vi "Image Data (Raw).vi"(8 "error in (no error)":errorcluster, 11 "Buffer in":refnum<class "Buffer.lvclass">=refnum) -> (0 "error out":errorcluster, 2 "Raw Data":string, 3 "Buffer":refnum<class "Buffer.lvclass">)   [LabVIEW 2020, in "common.lvlib" / "Buffer.lvclass"]
uses:
  Buffer.lvclass
  bin/gindustrialcam_32-1.dll
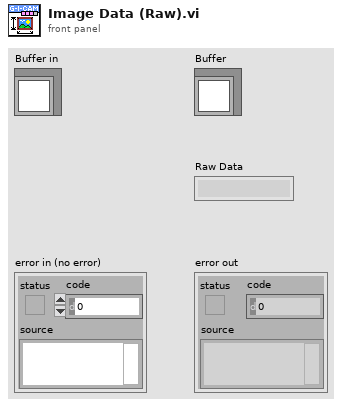
[diagram p1: front panel]
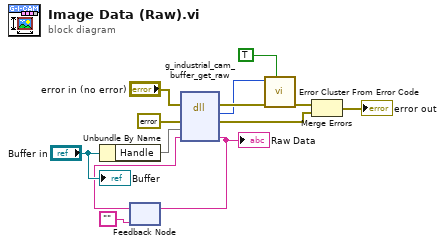
[diagram p0: block diagram]
diagram:
  n1 = Unbundle By Name("Buffer in") -> ("Handle"=w6)
  n2 = feedback #1("") -> (w1:string)
  n3 = dll-call lib="C:/Workspace/SSDC/g-industrial-camera/LabVIEW/g_industrial_cam/bin/gindustrialcam_*-1.*" fn="g_industrial_cam_buffer_get_raw"(error in="error in (no error)", "err"=errorcluster {"status"=FALSE, "code"=0, "source"=""} ("error constant"), "edvr"=w6, "data"=w1) -> (error out=w12:errorcluster, "Mg_Error"=w11:i32, "err"=w9:errorcluster, "data"=w2:string)  [unwired: 3 in, 1 out]
  "Raw Data" <- w2
  n4 = feedback-in #1(w2) -> ()
  n5 = call <vilib>:"Error Cluster From Error Code.vi"("show call chain? (False)"=TRUE, "error in (no error)"=w12, "error code (0)"=w11) -> ("error out"=w10:errorcluster)  [unwired: 6 in]
  n6 = Merge Errors(w10, w9) -> (→"error out":errorcluster)
  "Buffer" <- "Buffer in"
